vi "ReadLogitech-controller.vi"() -> ()   [LabVIEW 2018]
uses:
  <vilib>/Utility/inputDevices.llb/joystickAcquire.vi
panel:
  out "cluster":T1
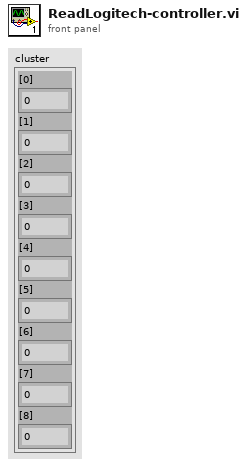
[diagram p1: front panel]
types:
  T1 = cluster{"[0]":dbl, "[1]":dbl, "[2]":dbl, "[3]":dbl, "[4]":dbl, "[5]":dbl, "[6]":dbl, "[7]":dbl, "[8]":dbl}
  T2 = cluster{"X axis":i32, "Y axis":i32, "Z axis":i32, "X axis rotation":i32, "Y axis rotation":i32, "Z axis rotation":i32, "U axis":i32, "V axis":i32}
  T3 = cluster{"Z axis":i32, "Z axis rotation":i32, i32, i32, i32, i32, i32, i32}
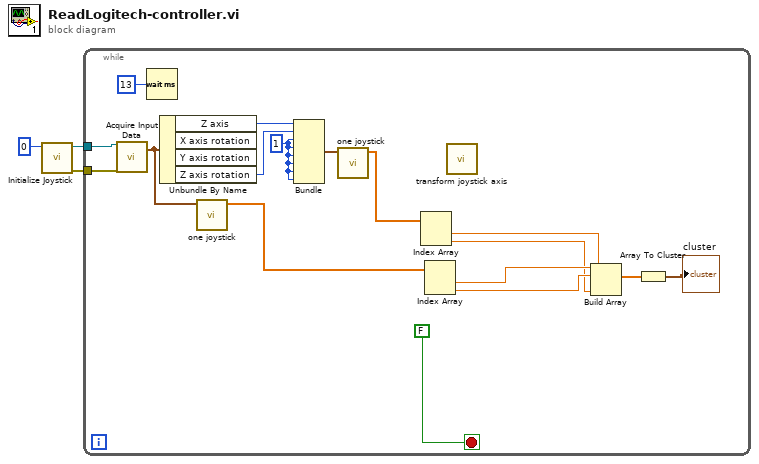
[diagram p0: block diagram]
diagram:
  n1 = call <vilib>:"Initialize Joystick.vi"("device index"=0) -> ("error out"=w2:errorcluster, "device ID"=w3:refnum<k1>)  [unwired: 9 in]
  n2 = while {
    tunnel: w3 -> [w19]
    tunnel: w2 -> [w18]
    stop <- FALSE stop-if-true
    w12 = 1
    n3 = call-poly <vilib>:"Acquire Input Data.vi"("device ID"=w19, "error in (no error)"=w18) -> ("axis info"=w16:T2)  [unwired: 13 in, 4 out]
    n4 = Wait (ms)(milliseconds to wait=u32 13) -> ()  [unwired: 1 out]
    n5 = Unbundle By Name(w16) -> ("Z axis"=w15:i32, "Z axis rotation"=w14:i32)  [unwired: 2 out]
    n6 = call <vilib>:"one joystick.vi"("axis info"=w16) -> ("Wheel Speeds [-1..1]"=w10:dbl[])  [unwired: 10 in]
    n7 = Bundle("Z axis"=w15, "Z axis rotation"=w14, w12, w12, w12, w12, w12, w12) -> (w13:T3)  [unwired: 1 in]
    n8 = call <vilib>:"one joystick.vi"("axis info"=w13) -> ("Wheel Speeds [-1..1]"=w11:dbl[])  [unwired: 10 in]
    n9 = Index Array(array=w11) -> (element #1=w5:dbl, element #2=w4:dbl)  [unwired: 2 in]
    n10 = Index Array(array=w10) -> (element #1=w9:dbl, element #2=w6:dbl)  [unwired: 2 in]
    n11 = call <vilib>:"transform joystick axis.vi"() -> ()  [unwired: 11 in, 1 out]
    n12 = Build Array(w9, w6, w5, w4) -> (w8:dbl[])
    n13 = Array To Cluster(array=w8) -> (cluster=→"cluster":T1)
  }
